vi "ScopeIntegrateSignal_Tdiag.vi"() -> ()   [LabVIEW 2018]
doc: "This example illustrates how to use autosetup and continuously acquires waveforms from a single channel using the following steps:\n\n1. Specify a valid VISA session. \n2. Specify a channel. \n3. Specify a time-out value for reading waveform.\n4. Run the VI. The graph displays the waveform you acquire."
uses:
  <vilib>/Analysis/8numeric.llb/1D Numeric Integration.vi
  <instrlib>/Tektronix DPO MSO 2000 4000 Series/Public/Data/Read (Multiple Waveforms).vi
  <vilib>/Waveform/WDTFileIO.llb/ Write Waveforms to File (1D).vi
  <instrlib>/Tektronix DPO MSO 2000 4000 Series/Tektronix DPO MSO 2000 4000 Series.lvlib
  <vilib>/Analysis/NI_AALPro.lvlib
panel:
  out "Savepath":path
  out "date/time string":string
  out "Waveform Data":waveform(dbl)[](graph)
  out "dt":dbl=4e-10
  out "error":i32
  out "integral (nVs)":dbl=768.7039999998229 format="%0.4f"
  out "stop int":dbl=2.580204778156997e-05
  out "start int":dbl=1.720136518771331e-05
  in  "Channel (0: Channel 1)":u16(ring)=1 items=["Channel 1", "Channel 2", "Channel 3", "Channel 4", "Math", "Reference 1", "Reference 2", "Reference 3", "Reference 4"]
  in  "Maximum Time (10000ms)":u32=10000
  in  "VISA Resource Name":refnum<visa-resource-name>="mdo4034c"
  out "Waveform Graph":waveform(dbl)(graph)={"t0"=timestamp(-1.7095999999994227e-05 s since 1904-01-01), "dt"=4e-10, "Y"=array[100000 elements]}
  # "(C) 2006 - 2022. National Instruments Corporation. ALL RIGHTS RESERVED."
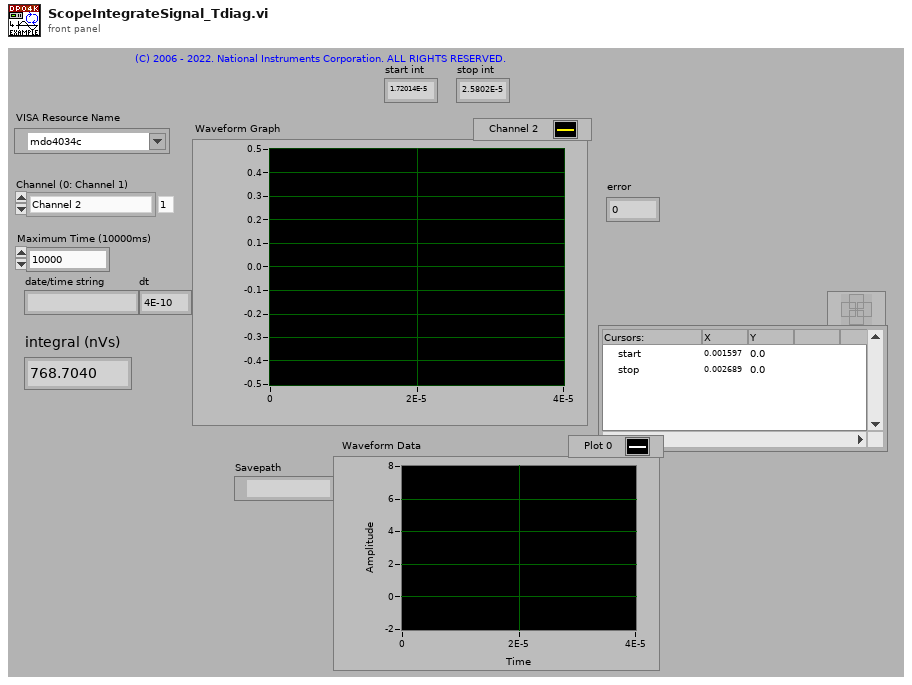
[diagram p1: front panel]
types:
  T1 = enum16{"open", "replace", "create", "open or create", "replace or create", "replace or create with confirmation"}
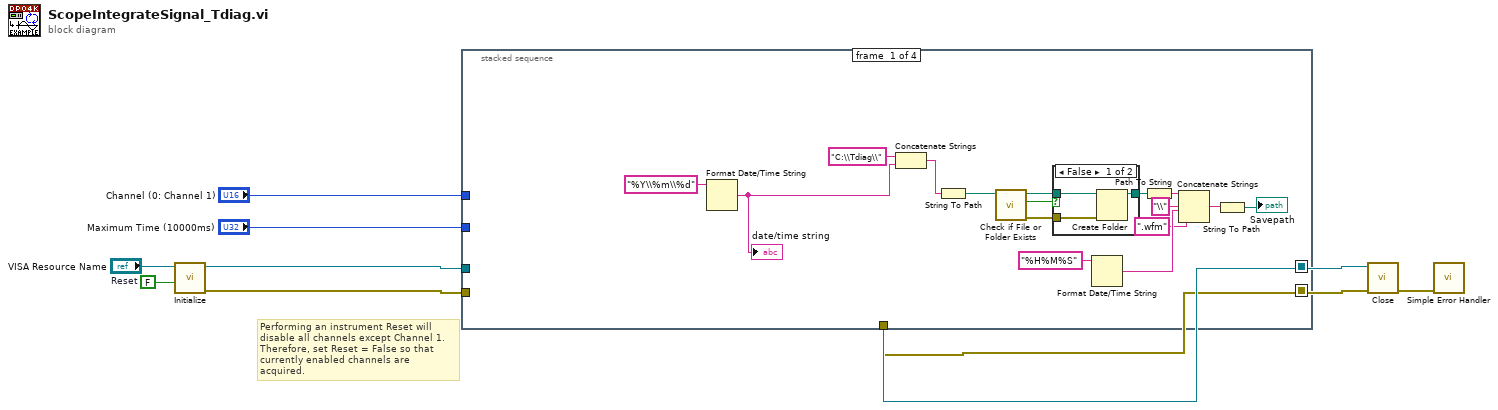
[diagram p0: block diagram]
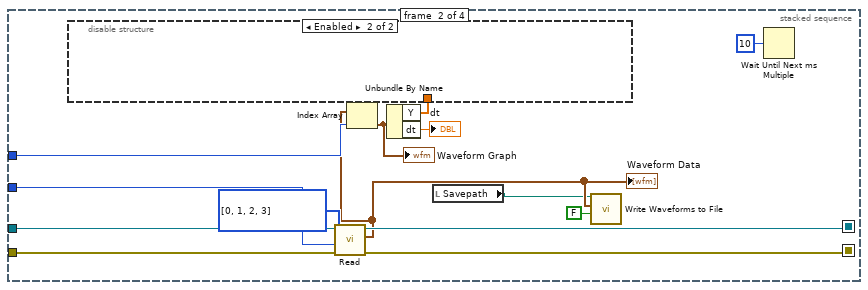
[diagram p3: hidden frame]
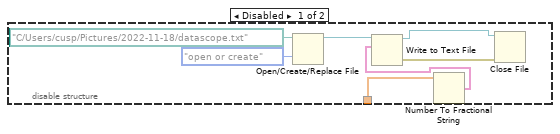
[diagram p4: hidden frame]
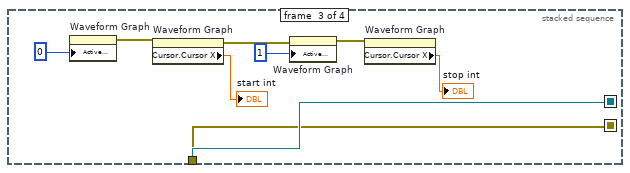
[diagram p5: hidden frame]
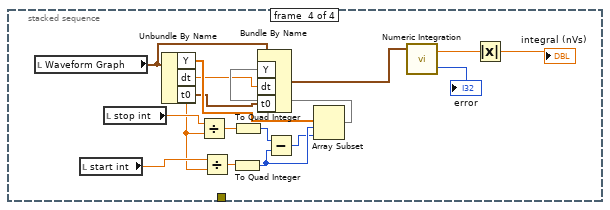
[diagram p6: hidden frame]
diagram:
  w5 = FALSE  # Reset
  # "Performing an instrument Reset will disable all channels except Channel 1. Therefore, set Reset = False so that currently enabled channels are acquired."
  n1 = call <instrlib>:"Initialize.vi"("Reset (True)"=w5, "VISA resource name"="VISA Resource Name") -> ("error out"=w2:errorcluster, "VISA resource name out"=w1:refnum<visa-resource-name>)  [unwired: 8 in]
  n2 = stacked-sequence {
    seq-local: [_ w41 _ _] -> [_ _ w59 _]
    seq-local: [_ w39 _ _] -> [_ _ w58 _]
    tunnel: w1 -> [_ w43 _ _]
    tunnel: w2 -> [_ w42 _ _]
    tunnel: "Maximum Time (10000ms)" -> [_ w38 _ _]
    tunnel: "Channel (0: Channel 1)" -> [_ w33 _ _]
    tunnel: [_ _ w59 _] -> w8
    tunnel: [_ _ w58 _] -> w7
    frame #0 {
      n3 = Format Date/Time String(time format string (%c)="%Y\\%m\\%d") -> (date/time string=w23:string)  [unwired: 2 in]
      "date/time string" <- w23
      n4 = Concatenate Strings("C:\\Tdiag\\" ("string"), w23) -> (w22:string)
      n5 = String To Path(string=w22) -> (path=w21:path)
      n6 = call <vilib>:"Check if File or Folder Exists.vi"("path"=w21) -> ("error out"=w18:errorcluster, "file or folder exists?"=w20:bool, "dup path"=w19:path)  [unwired: 8 in]
      n7 = case shown="False" w20 {
        tunnel: w19 -> [w28 w29]
        tunnel: w18 -> [w27 _]
        tunnel: [w26 w29] -> w17
        frame False {
          n8 = Create Folder(path (use dialog)=w28, error in=w27) -> (created path=w26:path)  [unwired: 1 in, 2 out]
        }
        frame True {
        }
      }
      n9 = Format Date/Time String(time format string (%c)="%H%M%S") -> (date/time string=w14:string)  [unwired: 2 in]
      n10 = Path To String(path=w17) -> (string=w16:string)
      n11 = Concatenate Strings(w16, "\\" ("string"), w14, ".wfm" ("string")) -> (w11:string)
      n12 = String To Path(string=w11) -> (path=→"Savepath":path)
    }
    frame #1 {
      w34 = u16[] [0, 1, 2, 3] items=["Channel 1", "Channel 2", "Channel 3", "Channel 4", "Math", "Reference 1", "Reference 2", "Reference 3", "Reference 4", "D0", "D1", "D2", "D3", "D4", "D5", "D6", "D7", "D8", "D9", "D10", "D11", "D12", "D13", "D14", "D15", "Amplitude", "Frequency", "Phase", "Normal", "Average", "Maximum Peak Hold", "Minimum Peak Hold"] ("Channels")
      n13 = call-poly <instrlib>:"Read.vi"("error in (no error)"=w42, "Maximum Time (10000ms)"=w38, "Channels"=w34, "VISA resource name"=w43) -> ("error out"=w39:errorcluster, "Waveform Data"=w32:waveform(dbl)[], "VISA resource name out"=w41:refnum<visa-resource-name>)  [unwired: 5 in]
      "Waveform Data" <- w32
      n14 = Index Array(array=w32, index=w33) -> (element=w35:waveform(dbl))
      "Waveform Graph" <- w35
      n15 = Unbundle By Name(w35) -> ("Y"=w36:dbl[], "dt"=→"dt":dbl)
      n16 = disable-structure shown="Enabled" {
        disable-tunnel: w36 -> [w48 _]
        frame Disabled {
          n17 = Open/Create/Replace File(file path (use dialog)=path "C:/Users/cusp/Pictures/2022-11-18/datascope.txt", operation (0:open)=T1."open or create") -> (refnum out=w49:refnum<file>)  [unwired: 4 in, 2 out]
          n18 = Number To Fractional String(number=w48) -> (F-format string=w47:string[])  [unwired: 3 in]
          n19 = Write to Text File(file (use dialog)=w49, text=w47) -> (refnum out=w46:refnum<file>, error out=w45:errorcluster)  [unwired: 2 in, 1 out]
          n20 = Close File(refnum=w46, error in=w45) -> ()  [unwired: 2 out]
        }
        frame Enabled {
        }
      }
      n21 = local read "Savepath"() -> (w30:path)
      n22 = call-poly <vilib>:"Write Waveforms to File.vi"("append to file? (new file:F)"=FALSE, "waveform array"=w32, "file path (dialog if empty)"=w30) -> ()  [unwired: 7 in, 2 out]
      n23 = Wait Until Next ms Multiple(millisecond multiple=u32 10) -> ()  [unwired: 1 out]
    }
    frame #2 {
      n24 = property on="Waveform Graph" class="WFGraph (strict)"("Active Cursor"=0 ("Cursor.Cursor Index")) -> (error out=w56:errorcluster)  [unwired: 2 in, 1 out]
      n25 = property on="Waveform Graph" class="WFGraph (strict)"(error in=w56) -> (error out=w55:errorcluster, "Cursor.Cursor X"=→"start int":dbl)  [unwired: 1 in, 1 out]
      n26 = property on="Waveform Graph" class="WFGraph (strict)"(error in=w55, "Active Cursor"=1 ("Cursor.Cursor Index")) -> (error out=w54:errorcluster)  [unwired: 1 in, 1 out]
      n27 = property on="Waveform Graph" class="WFGraph (strict)"(error in=w54) -> ("Cursor.Cursor X"=→"stop int":dbl)  [unwired: 1 in, 2 out]
    }
    frame #3 {
      n28 = local read "Waveform Graph"() -> (w66:waveform(dbl))
      n29 = local read "start int"() -> (w74:dbl)
      n30 = local read "stop int"() -> (w75:dbl)
      n31 = Unbundle By Name(w66) -> ("Y"=w64:dbl[], "dt"=w63:dbl, "t0"=w62:timestamp)
      n32 = Divide(x=w75, y=w63) -> (x/y=w73:dbl)
      n33 = Divide(x=w74, y=w63) -> (x/y=w72:dbl)
      n34 = To Quad Integer(1:w72) -> (0:w70:i64)
      n35 = To Quad Integer(1:w73) -> (0:w71:i64)
      n36 = Subtract(x=w71, y=w70) -> (x-y=w69:i64)
      n37 = Array Subset(array=w64, index=w70, length=w69) -> (w65:dbl[])
      n38 = Bundle By Name(cluster=w66, "Y"=w65, "dt"=w63, "t0"=w62) -> (w61:waveform(dbl))
      n39 = call-poly <vilib>:"Numeric Integration.vi"("Input Array"=w61) -> ("error"=→"error":i32, "result"=w68:dbl)  [unwired: 2 in]
      n40 = Absolute Value(x=w68) -> (abs(x)=→"integral (nVs)":dbl)
    }
  }
  n41 = call <instrlib>:"Close.vi"("error in (no error)"=w7, "VISA resource name"=w8) -> ("error out"=w6:errorcluster)  [unwired: 9 in]
  n42 = call <vilib>:"Simple Error Handler.vi"("error in (no error)"=w6) -> ()  [unwired: 4 in, 5 out]
